vi "TTLTrackercalc_171213.vi"(6 "Outside in":dbl[](array[numeric]), 9 "Inside in":dbl[](array[numeric]), 10 "Boolean":bool, 11 "MATCH index":i32) -> (0 "TTLduration":i32, 2 "Inside out":dbl[](array[numeric]), 3 "Outside out":dbl[](array[numeric]))   [LabVIEW 2016]
uses:
  Globaltracker.vi
panel:
  in  "TTLstaying":bool
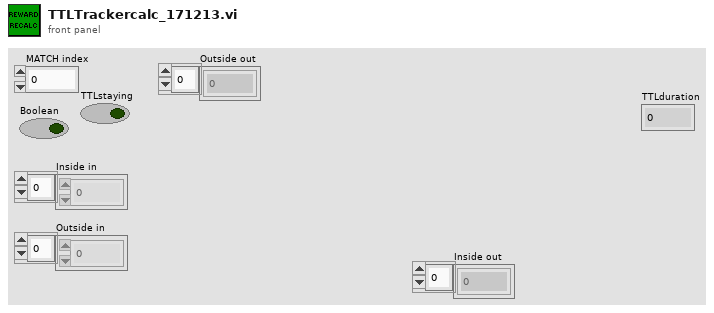
[diagram p1: front panel]
types:
  T1 = cluster{"Region number":i32, "ON/OFF":bool, "Activation type":string, "Activation critaria":i32, "Reward":i32}[]
  T2 = cluster{"Region number":i32, "ON/OFF":bool, "Activation type":string, "Activation critaria":i32, "Reward":i32}
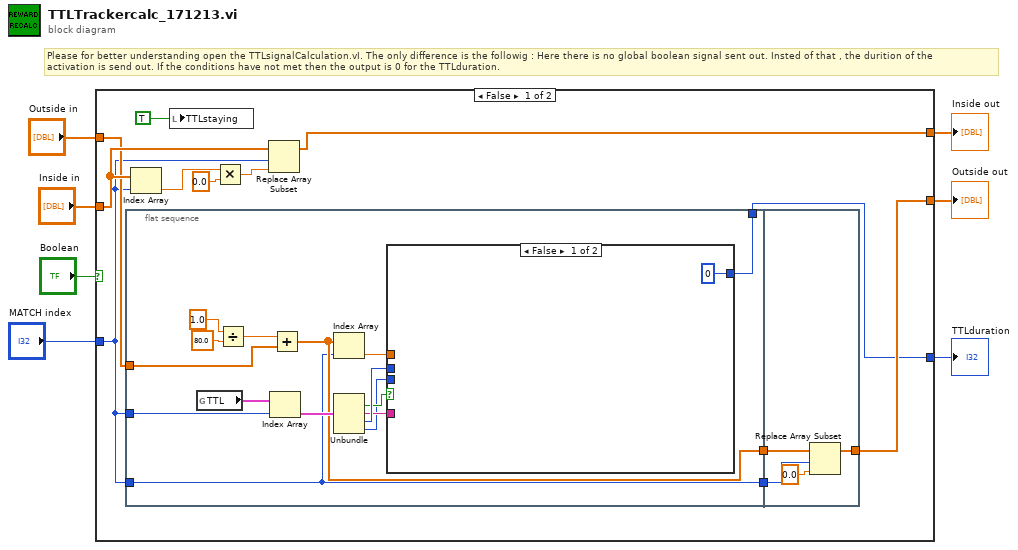
[diagram p0: block diagram]
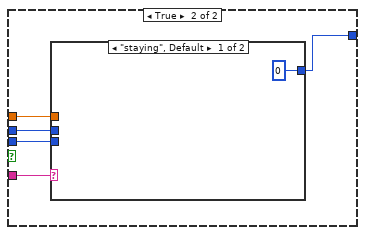
[diagram p2: hidden frame]
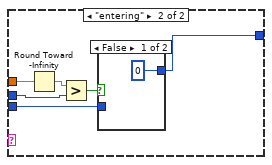
[diagram p3: hidden frame]
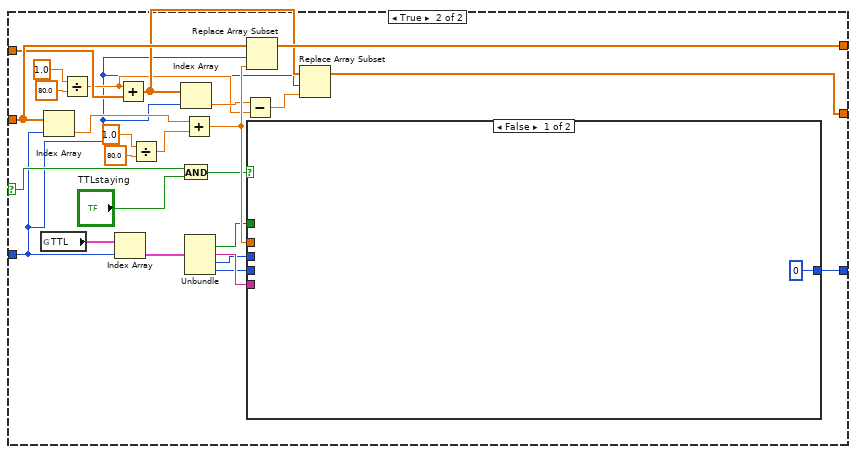
[diagram p5: hidden frame]
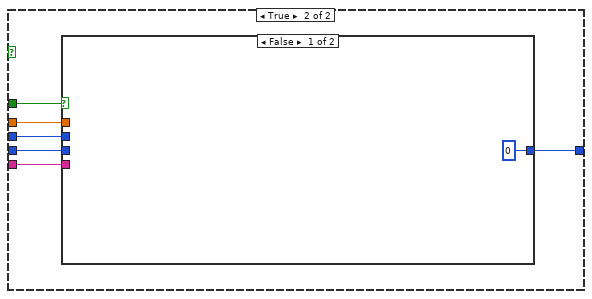
[diagram p6: hidden frame]
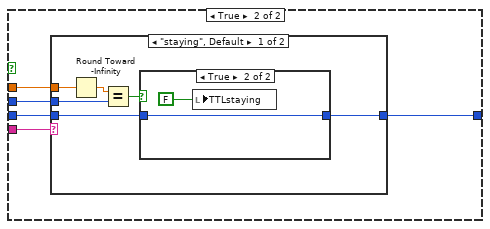
[diagram p7: hidden frame]
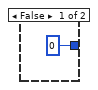
[diagram p8: hidden frame]
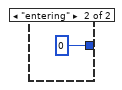
[diagram p9: hidden frame]
diagram:
  # "Please for better understanding open the TTLsignalCalculation.vI. The only difference is the followig : Here there is no global boolean signal sent out. Insted of that , the durition of the \nactivation is send out. If the conditions have not met then the output is 0 for the TTLduration."
  n1 = case shown="False" "Boolean" {
    selector: "Boolean" -> [_ w64]
    tunnel: "Inside in" -> [w17 w74]
    tunnel: [w15 w75] -> w3
    tunnel: "MATCH index" -> [w10 w60]
    tunnel: "Outside in" -> [w12 w66]
    tunnel: [w11 w67] -> w5
    tunnel: [w8 w54] -> w1
    frame False {
      n2 = flat-sequence {
        tunnel: w12 -> [w26]
        tunnel: w10 -> [w23]
        tunnel: [w25] -> w14
        tunnel: [w23] -> w13
        tunnel: w10 -> [w22]
        tunnel: [w20] -> w8
        tunnel: w14 -> [w52]
        tunnel: w13 -> [w51]
        tunnel: [w53] -> w11
        frame #0 {
          n3 = global read "Globaltracker.vi" "TTL"() -> (w34:T1)
          n4 = Divide(x=1.0, y=80.0) -> (x/y=w27:dbl)
          n5 = Index Array(array=w34, index=w22) -> (element=w30:T2)
          n6 = Add(x=w27, y=w26) -> (x+y=w25:dbl[])
          n7 = Index Array(array=w25, index=w23) -> (element=w24:dbl)
          n8 = Unbundle(w30) -> ("ON/OFF"=w31:bool, "Activation type"=w32:string, "Activation critaria"=w33:i32, "Reward"=w21:i32)  [unwired: 1 out]
          n9 = case shown="False" w31 {
            tunnel: w32 -> [_ w40]
            tunnel: w33 -> [_ w39]
            tunnel: w24 -> [_ w38]
            tunnel: w21 -> [_ w37]
            tunnel: [0 ("Reward") w36] -> w20
            frame False {
            }
            frame True {
              n10 = case shown="\"staying\", Default" w40 {
                tunnel: w39 -> [_ w44]
                tunnel: w38 -> [_ w45]
                tunnel: w37 -> [_ w43]
                tunnel: [0 ("Reward") w42] -> w36
                frame "staying", Default {
                }
                frame "entering" {
                  n11 = Round Toward -Infinity(1:w45) -> (0:w46:dbl)
                  n12 = Greater?(x=w46, y=w44) -> (0:w47:bool)
                  n13 = case shown="False" w47 {
                    tunnel: w43 -> [_ w49]
                    tunnel: [0 ("Reward") w49] -> w42
                    frame False {
                    }
                    frame True {
                    }
                  }
                }
              }
            }
          }
        }
        frame #1 {
          n14 = Replace Array Subset(array=w52, new element=0.0 ("new element/subarray"), index=w51) -> (w53:dbl[])
        }
      }
      n15 = Index Array(array=w17, index=w10) -> (element=w18:dbl)
      n16 = local write "TTLstaying"(TRUE ("reward staying")) -> ()
      n17 = Multiply(x=w18, y=0.0) -> (x*y=w19:dbl)
      n18 = Replace Array Subset(array=w17, new element=w19, index=w10) -> (w15:dbl[])
    }
    frame True {
      n19 = global read "Globaltracker.vi" "TTL"() -> (w62:T1)
      n20 = Index Array(array=w74, index=w60) -> (element=w76:dbl)
      n21 = Divide(x=1.0, y=80.0) -> (x/y=w65:dbl)
      n22 = Index Array(array=w62, index=w60) -> (element=w61:T2)
      n23 = Add(x=w65, y=w66) -> (x+y=w70:dbl[])
      n24 = Divide(x=1.0, y=80.0) -> (x/y=w77:dbl)
      n25 = Index Array(array=w70, index=w60) -> (element=w71:dbl)
      n26 = And(x=w64, y="TTLstaying") -> (x .and. y?=w63:bool)
      n27 = Add(x=w76, y=w77) -> (x+y=w73:dbl)
      n28 = Unbundle(w61) -> ("ON/OFF"=w59:bool, "Activation type"=w58:string, "Activation critaria"=w57:i32, "Reward"=w55:i32)  [unwired: 1 out]
      n29 = Subtract(x=w71, y=w65) -> (x-y=w72:dbl)
      n30 = Replace Array Subset(array=w74, new element=w73, index=w60) -> (w75:dbl[])
      n31 = case shown="False" w63 {
        tunnel: w73 -> [_ w86]
        tunnel: w59 -> [_ w85]
        tunnel: w58 -> [_ w84]
        tunnel: w57 -> [_ w83]
        tunnel: w55 -> [_ w82]
        tunnel: [0 ("Reward") w81] -> w54
        frame False {
        }
        frame True {
          n32 = case shown="False" w85 {
            tunnel: w86 -> [_ w92]
            tunnel: w84 -> [_ w91]
            tunnel: w83 -> [_ w90]
            tunnel: w82 -> [_ w89]
            tunnel: [0 ("Reward") w88] -> w81
            frame False {
            }
            frame True {
              n33 = case shown="\"staying\", Default" w91 {
                tunnel: w92 -> [w98 _]
                tunnel: w90 -> [w95 _]
                tunnel: w89 -> [w94 _]
                tunnel: [w93 0 ("Reward")] -> w88
                frame "staying", Default {
                  n34 = Round Toward -Infinity(1:w98) -> (0:w96:dbl)
                  n35 = Equal?(x=w96, y=w95) -> (x = y?=w97:bool)
                  n36 = case shown="True" w97 {
                    tunnel: w94 -> [_ w101]
                    tunnel: [0 ("Reward") w101] -> w93
                    frame False {
                    }
                    frame True {
                      n37 = local write "TTLstaying"(FALSE ("reward staying")) -> ()
                    }
                  }
                }
                frame "entering" {
                }
              }
            }
          }
        }
      }
      n38 = Replace Array Subset(array=w70, new element=w72, index=w60) -> (w67:dbl[])
    }
  }
  "Outside out" <- w5
  "Inside out" <- w3
  "TTLduration" <- w1
